vi "Msg Loop.vi"(11 "Actor in":refnum<class "LVCAM.lvclass">) -> ()   [LabVIEW 2021, in "AAM.lvlib" / "LVCAM.lvclass"]
uses:
  LVCAM.lvclass
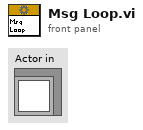
[diagram p1: front panel]
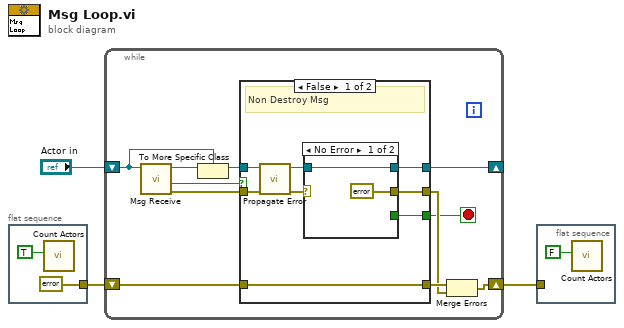
[diagram p0: block diagram]
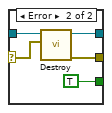
[diagram p2: hidden frame]
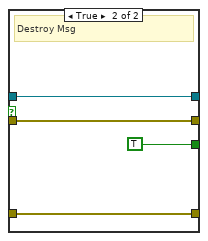
[diagram p3: hidden frame]
diagram:
  n1 = flat-sequence {
    tunnel: [errorcluster {"status"=FALSE, "code"=0, "source"=""} ("error out")] -> w2
    frame #0 {
      n2 = call "Count Actors.vi"("Increment?"=TRUE) -> ()  [unwired: 11 in]
    }
  }
  n3 = while {
    shift-right: [w16] -> _
    shift-left: "Actor in" -> [w13]
    shift-right: [w9] -> w1
    shift-left: w2 -> [w11]
    stop <- w7 stop-if-true
    n4 = call-dynamic "Msg Receive.vi"("Msg Receive in"=w13) -> ("error out"=w10:errorcluster, "Destroy Self?"=w6:bool, "Msg Receive out"=w15:refnum<class "Msg Receive.lvclass">)  [unwired: 8 in]
    n5 = To More Specific Class(target class=w13, reference=w15) -> (specific class reference=w14:refnum<class "LVCAM.lvclass">)  [unwired: 1 in, 1 out]
    n6 = case shown="False" w6 {
      tunnel: w10 -> [w21 w33]
      tunnel: [w24 w35] -> w16
      tunnel: w14 -> [w22 w35]
      tunnel: [w23 TRUE] -> w7
      tunnel: [w18 w34] -> w12
      tunnel: w11 -> [w18 w34]
      tunnel: [w17 w33] -> w8
      frame False {
        # "Non Destroy Msg"
        n7 = call-dynamic "Propagate Error.vi"("error in (no error)"=w21, "Propagate Error in"=w22) -> ("error out"=w19:errorcluster, "Propagate Error out"=w20:refnum<class "LVCAM.lvclass">)  [unwired: 8 in]
        n8 = case shown="No Error" w19 {
          selector: w19 -> [_ w28]
          tunnel: [w26 w29] -> w24
          tunnel: w20 -> [w26 w30]
          tunnel: [_ TRUE] -> w23
          tunnel: [errorcluster {"status"=FALSE, "code"=0, "source"=""} ("error out") w27] -> w17
          frame No Error {
          }
          frame Error {
            n9 = call-dynamic "Destroy.vi"("Error"=w28, "Destroy in"=w30) -> ("error out"=w27:errorcluster, "Destroy out"=w29:refnum<class "LVCAM.lvclass">)  [unwired: 8 in]
          }
        }
      }
      frame True {
        # "Destroy Msg"
      }
    }
    n10 = Merge Errors(w12, w8) -> (w9:errorcluster)
  }
  n11 = flat-sequence {
    tunnel: w1 -> [_]
    frame #0 {
      n12 = call "Count Actors.vi"("Increment?"=FALSE) -> ()  [unwired: 11 in]
    }
  }
